vi "AddPara.vi"(8 "error in":errorcluster caption="错误输入", 10 "选择":enum16{"上报时间", "电池类型", "软件版本"}(ring), 11 "Setup":T1) -> (0 "error out":errorcluster caption="错误输出")   [LabVIEW 2013]
uses:
  SetupCtl.ctl
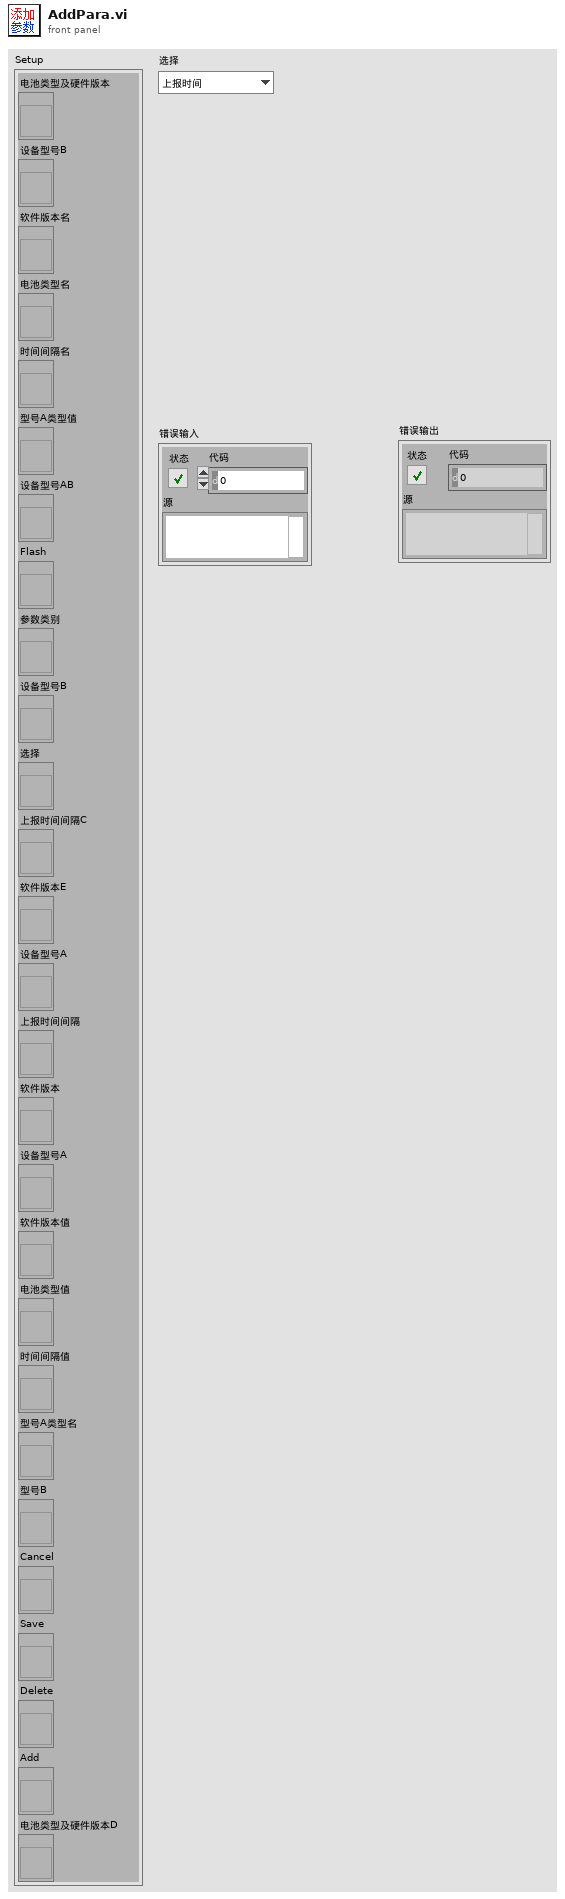
[diagram p1: front panel]
types:
  T1 = typedef "SetupCtl.ctl" = cluster{"电池类型及硬件版本":refnum<vi>, "设备型号B":refnum<vi>, "软件版本名":refnum<vi>, "电池类型名":refnum<vi>, "时间间隔名":refnum<vi>, "型号A类型值":refnum<vi>, "设备型号AB":refnum<vi>, "Flash":refnum<vi>, "参数类别":refnum<vi>, "设备型号B":refnum<vi>, "选择":refnum<vi>, "上报时间间隔C":refnum<vi>, "软件版本E":refnum<vi>, "设备型号A":refnum<vi>, "上报时间间隔":refnum<vi>, "软件版本":refnum<vi>, "设备型号A":refnum<vi>, "软件版本值":refnum<vi>, "电池类型值":refnum<vi>, "时间间隔值":refnum<vi>, "型号A类型名":refnum<vi>, "型号B":refnum<vi>, "Cancel":refnum<vi>, "Save":refnum<vi>, "Delete":refnum<vi>, "Add":refnum<vi>, "电池类型及硬件版本D":refnum<vi>}
  T2 = enum16{"型号AB", "型号A", "型号B", "上报时间间隔", "电池类型", "软件版本"}
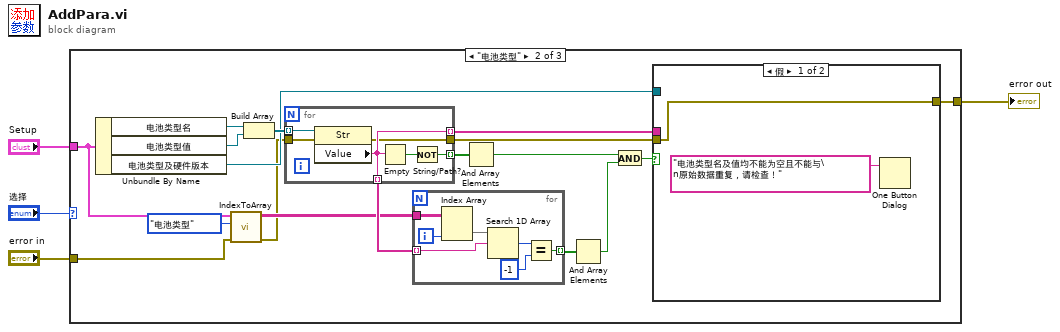
[diagram p0: block diagram]
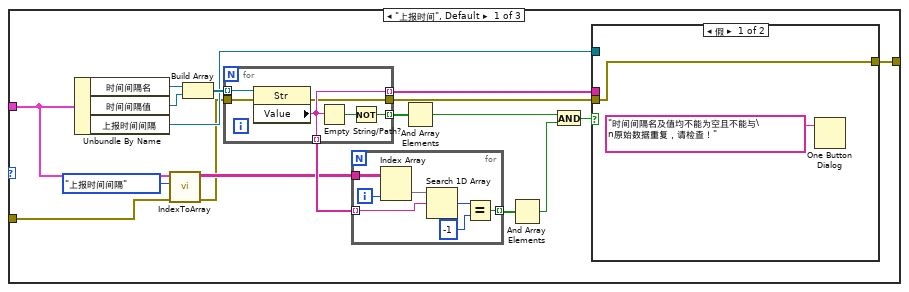
[diagram p2: hidden frame]
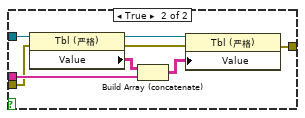
[diagram p3: hidden frame]
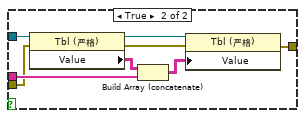
[diagram p4: hidden frame]
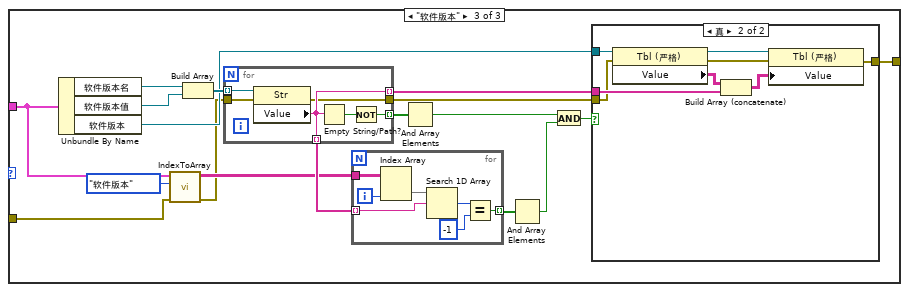
[diagram p5: hidden frame]
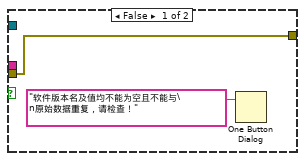
[diagram p6: hidden frame]
diagram:
  n1 = case shown="\"电池类型\"" "选择" {
    tunnel: "Setup" -> [w18 w59 w100]
    tunnel: "error in" -> [w8 w49 w90]
    tunnel: [w5 w46 w87] -> w1
    frame "上报时间", Default {
      n2 = Unbundle By Name(w18) -> ("时间间隔名"=w22:refnum<vi>, "时间间隔值"=w21:refnum<vi>, "上报时间间隔"=w10:refnum<vi>)
      n3 = call "IndexToArray.vi"("error in"=w8, "Extract"=T2."上报时间间隔", "Setup"=w18) -> ("error out"=w7:errorcluster, "Value"=w15:string[][])  [unwired: 7 in]
      n4 = Build Array(w22, w21) -> (w20:refnum<vi>[])
      n5 = for {
        tunnel: w20 -> [w45] mode=indexing
        tunnel: [w43] -> w19 mode=indexing
        tunnel: [w42] -> w16 mode=indexing
        tunnel: [w42] -> w9 mode=indexing
        tunnel: w7 -> [w41]
        tunnel: [w40] -> w6
        n6 = property class="Str"(reference=w45, error in=w41) -> (error out=w40:errorcluster, "Value"=w42:string)  [unwired: 1 out]
        n7 = Empty String/Path?(string/path=w42) -> (empty?=w44:bool)
        n8 = Not(x=w44) -> (.not. x?=w43:bool)
      }
      n9 = for {
        tunnel: w16 -> [w36] mode=indexing
        tunnel: w15 -> [w39]
        tunnel: [w33] -> w14 mode=indexing
        i -> [w38]
        n10 = Index Array(array=w39, index (col)=w38) -> (element=w37:string[])  [unwired: 1 in]
        n11 = Search 1D Array(1D array=w37, element=w36) -> (index of element=w35:i32)  [unwired: 1 in]
        n12 = Equal?(x=w35, y=-1) -> (x = y?=w33:bool)
      }
      n13 = And Array Elements(Boolean array=w19) -> (logical AND=w13:bool)
      n14 = And Array Elements(Boolean array=w14) -> (logical AND=w12:bool)
      n15 = And(x=w13, y=w12) -> (x .and. y?=w11:bool)
      n16 = case shown="假" w11 {
        tunnel: w10 -> [_ w32]
        tunnel: w9 -> [_ w30]
        tunnel: w6 -> [w24 w27]
        tunnel: [w24 w25] -> w5
        frame False {
          n17 = One Button Dialog(message="时间间隔名及值均不能为空且不能与\n原始数据重复，请检查！" ("消息")) -> ()  [unwired: 1 in, 1 out]
        }
        frame True {
          n18 = property class="Tbl (严格)"(reference=w32, error in=w27) -> (reference out=w28:refnum<vi>, error out=w26:errorcluster, "Value"=w31:string[][])
          n19 = Build Array (concatenate)(w31, w30) -> (w29:string[][])
          n20 = property class="Tbl (严格)"(reference=w28, error in=w26, "Value"=w29) -> (error out=w25:errorcluster)  [unwired: 1 out]
        }
      }
    }
    frame "电池类型" {
      n21 = Unbundle By Name(w59) -> ("电池类型名"=w63:refnum<vi>, "电池类型值"=w62:refnum<vi>, "电池类型及硬件版本"=w51:refnum<vi>)
      n22 = call "IndexToArray.vi"("error in"=w49, "Extract"=T2."电池类型", "Setup"=w59) -> ("error out"=w48:errorcluster, "Value"=w56:string[][])  [unwired: 7 in]
      n23 = Build Array(w63, w62) -> (w61:refnum<vi>[])
      n24 = for {
        tunnel: w61 -> [w86] mode=indexing
        tunnel: [w84] -> w60 mode=indexing
        tunnel: [w83] -> w57 mode=indexing
        tunnel: [w83] -> w50 mode=indexing
        tunnel: w48 -> [w82]
        tunnel: [w81] -> w47
        n25 = property class="Str"(reference=w86, error in=w82) -> (error out=w81:errorcluster, "Value"=w83:string)  [unwired: 1 out]
        n26 = Empty String/Path?(string/path=w83) -> (empty?=w85:bool)
        n27 = Not(x=w85) -> (.not. x?=w84:bool)
      }
      n28 = for {
        tunnel: w57 -> [w77] mode=indexing
        tunnel: w56 -> [w80]
        tunnel: [w74] -> w55 mode=indexing
        i -> [w79]
        n29 = Index Array(array=w80, index (col)=w79) -> (element=w78:string[])  [unwired: 1 in]
        n30 = Search 1D Array(1D array=w78, element=w77) -> (index of element=w76:i32)  [unwired: 1 in]
        n31 = Equal?(x=w76, y=-1) -> (x = y?=w74:bool)
      }
      n32 = And Array Elements(Boolean array=w60) -> (logical AND=w54:bool)
      n33 = And Array Elements(Boolean array=w55) -> (logical AND=w53:bool)
      n34 = And(x=w54, y=w53) -> (x .and. y?=w52:bool)
      n35 = case shown="假" w52 {
        tunnel: w51 -> [_ w73]
        tunnel: w50 -> [_ w71]
        tunnel: w47 -> [w65 w68]
        tunnel: [w65 w66] -> w46
        frame False {
          n36 = One Button Dialog(message="电池类型名及值均不能为空且不能与\n原始数据重复，请检查！" ("消息")) -> ()  [unwired: 1 in, 1 out]
        }
        frame True {
          n37 = property class="Tbl (严格)"(reference=w73, error in=w68) -> (reference out=w69:refnum<vi>, error out=w67:errorcluster, "Value"=w72:string[][])
          n38 = Build Array (concatenate)(w72, w71) -> (w70:string[][])
          n39 = property class="Tbl (严格)"(reference=w69, error in=w67, "Value"=w70) -> (error out=w66:errorcluster)  [unwired: 1 out]
        }
      }
    }
    frame "软件版本" {
      n40 = Unbundle By Name(w100) -> ("软件版本名"=w104:refnum<vi>, "软件版本值"=w103:refnum<vi>, "软件版本"=w92:refnum<vi>)
      n41 = call "IndexToArray.vi"("error in"=w90, "Extract"=T2."软件版本", "Setup"=w100) -> ("error out"=w89:errorcluster, "Value"=w97:string[][])  [unwired: 7 in]
      n42 = Build Array(w104, w103) -> (w102:refnum<vi>[])
      n43 = for {
        tunnel: w102 -> [w127] mode=indexing
        tunnel: [w125] -> w101 mode=indexing
        tunnel: [w124] -> w98 mode=indexing
        tunnel: [w124] -> w91 mode=indexing
        tunnel: w89 -> [w123]
        tunnel: [w122] -> w88
        n44 = property class="Str"(reference=w127, error in=w123) -> (error out=w122:errorcluster, "Value"=w124:string)  [unwired: 1 out]
        n45 = Empty String/Path?(string/path=w124) -> (empty?=w126:bool)
        n46 = Not(x=w126) -> (.not. x?=w125:bool)
      }
      n47 = for {
        tunnel: w98 -> [w118] mode=indexing
        tunnel: w97 -> [w121]
        tunnel: [w115] -> w96 mode=indexing
        i -> [w120]
        n48 = Index Array(array=w121, index (col)=w120) -> (element=w119:string[])  [unwired: 1 in]
        n49 = Search 1D Array(1D array=w119, element=w118) -> (index of element=w117:i32)  [unwired: 1 in]
        n50 = Equal?(x=w117, y=-1) -> (x = y?=w115:bool)
      }
      n51 = And Array Elements(Boolean array=w101) -> (logical AND=w95:bool)
      n52 = And Array Elements(Boolean array=w96) -> (logical AND=w94:bool)
      n53 = And(x=w95, y=w94) -> (x .and. y?=w93:bool)
      n54 = case shown="真" w93 {
        tunnel: w92 -> [_ w114]
        tunnel: w91 -> [_ w112]
        tunnel: w88 -> [w106 w109]
        tunnel: [w106 w107] -> w87
        frame False {
          n55 = One Button Dialog(message="软件版本名及值均不能为空且不能与\n原始数据重复，请检查！" ("消息")) -> ()  [unwired: 1 in, 1 out]
        }
        frame True {
          n56 = property class="Tbl (严格)"(reference=w114, error in=w109) -> (reference out=w110:refnum<vi>, error out=w108:errorcluster, "Value"=w113:string[][])
          n57 = Build Array (concatenate)(w113, w112) -> (w111:string[][])
          n58 = property class="Tbl (严格)"(reference=w110, error in=w108, "Value"=w111) -> (error out=w107:errorcluster)  [unwired: 1 out]
        }
      }
    }
  }
  "error out" <- w1
